vi "energy_optimization_15.vi"() -> ()   [LabVIEW 2016]
uses:
  <vilib>/httpClient/LabVIEWHTTPClient.lvlib
panel:
  out "Battery Output":dbl
  in  "stop":bool
  out "Credits":dbl
  out "Solar+AC+Battery":dbl
  out "Battery":dbl
  in  "Illuminance":dbl
  out "ShutDown":bool
  out "Battery LED":bool
  out "AC LED":bool
  out "Solar LED":bool
  out "AC Output":dbl
  out "Solar Output":dbl
  out "Solar+AC":dbl
  out "Solar Voltage":dbl
  in  "Required":dbl
  out "DC Voltage":dbl
  out "Three Phase Signal":dynamicdata(graph)
  # "OUTPUTS"
  # "INPUTS"
  # "INTERMEDIATE STORAGE"
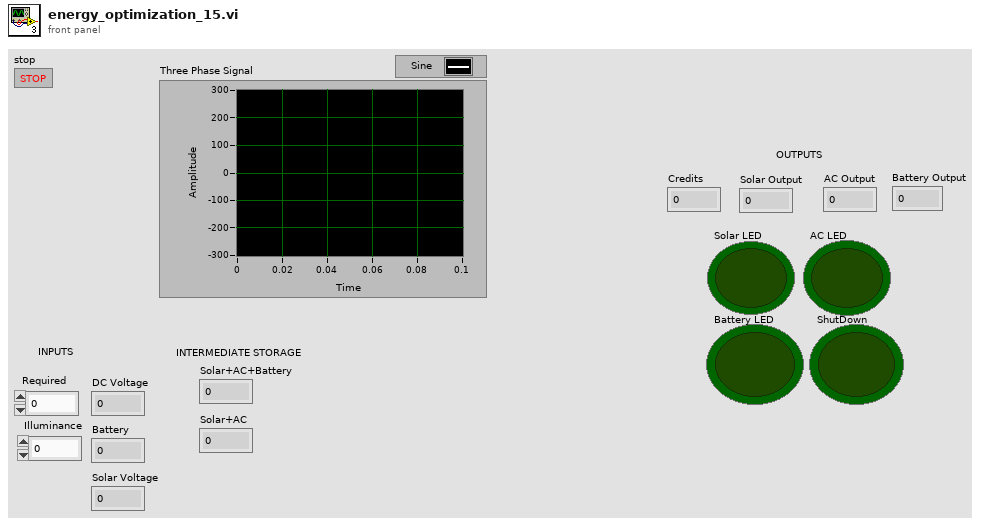
[diagram p1: front panel]
types:
  T1 = typedef "LabVIEWHTTPClient.lvlib/ClientHandle.ctl" = refnum<k1>
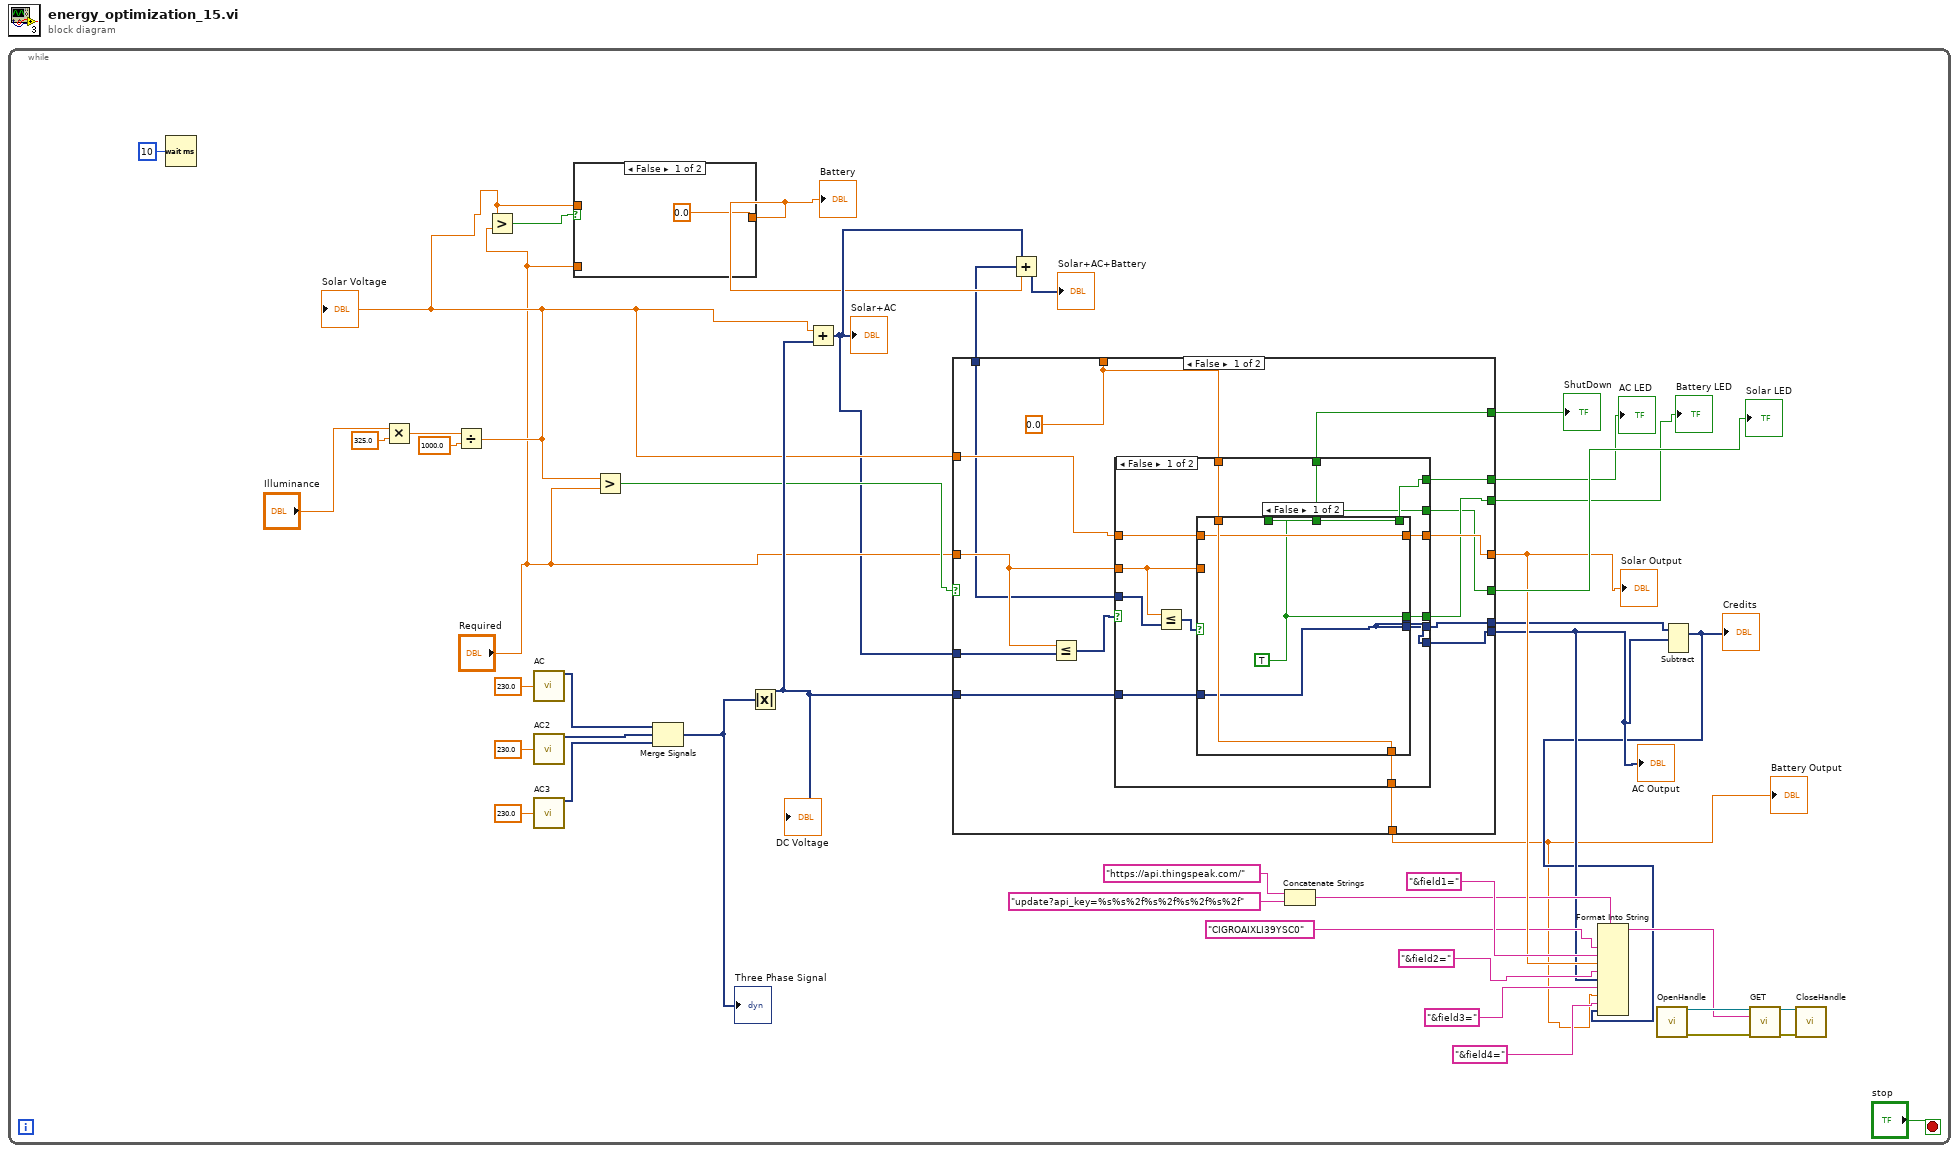
[diagram p0: block diagram]
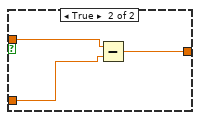
[diagram p2: hidden frame]
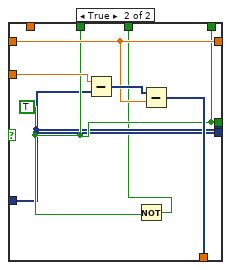
[diagram p3: hidden frame]
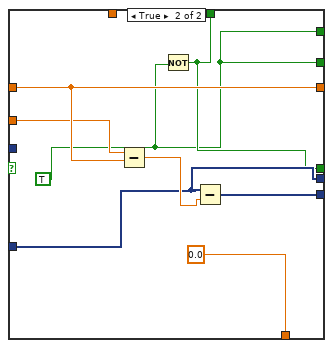
[diagram p4: hidden frame]
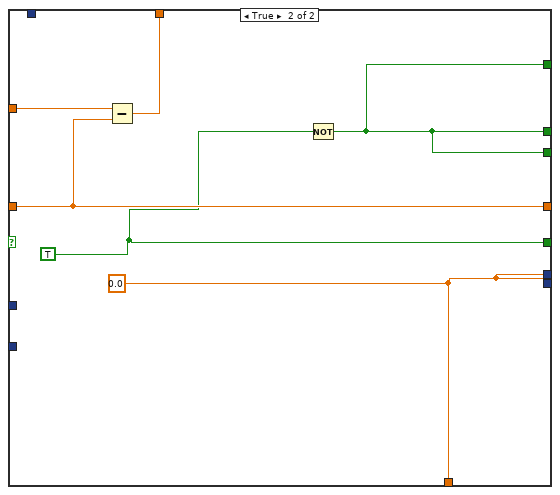
[diagram p5: hidden frame]
diagram:
  n1 = while {
    stop <- "stop" stop-if-true
    n2 = Wait (ms)(milliseconds to wait=u32 10) -> ()  [unwired: 1 out]
    n3 = Multiply(x="Illuminance", y=325.0) -> (x*y=w35:dbl)
    n4 = Divide(x=w35, y=1000.0) -> (x/y=w25:dbl)
    "Solar Voltage" <- w25
    n5 = Greater?(x=w25, y="Required") -> (0:w26:bool)
    n6 = call "AC"("Amplitude"=230.0) -> ("Sine"=w43:dynamicdata)  [unwired: 13 in, 1 out]
    n7 = call "AC2"("Amplitude"=230.0) -> ("Sine"=w42:dynamicdata)  [unwired: 13 in, 1 out]
    n8 = call "AC3"("Amplitude"=230.0) -> ("Sine"=w41:dynamicdata)  [unwired: 13 in, 1 out]
    n9 = case shown="False" w26 {
      tunnel: w25 -> [_ w47]
      tunnel: "Required" -> [_ w46]
      tunnel: [0.0 ("Amplitude") w45] -> w22
      frame False {
      }
      frame True {
        n10 = Subtract(x=w47, y=w46) -> (x-y=w45:dbl)
      }
    }
    "Battery" <- w22
    n11 = Greater?(x=w25, y="Required") -> (0:w28:bool)
    n12 = Merge Signals(w43, w42, w41) -> (w40:dynamicdata)
    "Three Phase Signal" <- w40
    n13 = Absolute Value(x=w40) -> (abs(x)=w29:dynamicdata)
    "DC Voltage" <- w29
    n14 = Add(x=w25, y=w29) -> (x+y=w23:dynamicdata)
    "Solar+AC" <- w23
    n15 = Add(x=w23, y=w22) -> (x+y=w21:dynamicdata)
    "Solar+AC+Battery" <- w21
    n16 = case shown="False" w28 {
      tunnel: [w56 w97] -> w7
      tunnel: [w55 w97] -> w1
      tunnel: [w51 w96] -> w33
      tunnel: [w52 w101] -> w32
      tunnel: [w50 w101] -> w31
      tunnel: [w53 w101] -> w30
      tunnel: w23 -> [w62 _]
      tunnel: "Required" -> [w58 w99]
      tunnel: [w59 w99] -> w12
      tunnel: w25 -> [w60 w100]
      tunnel: [w54 w98] -> _
      tunnel: w29 -> [w57 _]
      tunnel: w21 -> [w49 _]
      tunnel: [w48 w97] -> w6
      frame False {
        w54 = 0.0 ("Amplitude")
        n17 = Less Or Equal?(x=w58, y=w62) -> (x <= y?=w61:dynamicdata)
        n18 = case shown="False" w61 {
          tunnel: w60 -> [w74 w95]
          tunnel: [w73 w95] -> w59
          tunnel: w58 -> [w64 w94]
          tunnel: w57 -> [w75 w90]
          tunnel: [w76 w92] -> w56
          tunnel: [w71 0.0 ("Amplitude")] -> w55
          tunnel: w54 -> [w70 _]
          tunnel: [w67 w89] -> w53
          tunnel: [w69 w88] -> w52
          tunnel: [w68 w88] -> w51
          tunnel: [w66 w89] -> w50
          tunnel: w49 -> [w65 _]
          tunnel: [w63 w90] -> w48
          frame False {
            n19 = Less Or Equal?(x=w64, y=w65) -> (x <= y?=w72:dynamicdata)
            n20 = case shown="False" w72 {
              tunnel: [w77 w82] -> w76
              tunnel: w75 -> [w77 w82]
              tunnel: w74 -> [w79 w85]
              tunnel: [w79 w85] -> w73
              tunnel: w64 -> [_ w87]
              tunnel: [w80 w84] -> w71
              tunnel: w70 -> [w80 _]
              tunnel: [w78 w83] -> w69
              tunnel: [w78 w83] -> w68
              tunnel: [w78 w83] -> w67
              tunnel: [w78 w81] -> w66
              tunnel: [w77 w82] -> w63
              frame False {
                w78 = TRUE
              }
              frame True {
                w83 = TRUE
                n21 = Subtract(x=w87, y=w82) -> (x-y=w86:dynamicdata)
                n22 = Not(x=w83) -> (.not. x?=w81:bool)
                n23 = Subtract(x=w86, y=w85) -> (x-y=w84:dynamicdata)
              }
            }
          }
          frame True {
            w88 = TRUE
            n24 = Subtract(x=w94, y=w95) -> (x-y=w93:dbl)
            n25 = Not(x=w88) -> (.not. x?=w89:bool)
            n26 = Subtract(x=w90, y=w93) -> (x-y=w92:dynamicdata)
          }
        }
      }
      frame True {
        w96 = TRUE
        w97 = 0.0 ("Amplitude")
        n27 = Subtract(x=w100, y=w99) -> (x-y=w98:dbl)
        n28 = Not(x=w96) -> (.not. x?=w101:bool)
      }
    }
    "Solar Output" <- w12
    "AC Output" <- w7
    "Solar LED" <- w33
    "AC LED" <- w32
    "Battery LED" <- w30
    "ShutDown" <- w31
    "Battery Output" <- w1
    n29 = Concatenate Strings("https://api.thingspeak.com/" ("string"), "update?api_key=%s%s%2f%s%2f%s%2f%s%2f" ("string")) -> (w9:string)
    n30 = call <vilib>:"OpenHandle.vi"() -> ("client handle out"=w19:T1, "error out"=w18:errorcluster)  [unwired: 14 in]
    n31 = Subtract(1:w7, 2:w6) -> (0:w3:dynamicdata)  [unwired: 1 in, 1 out]
    "Credits" <- w3
    n32 = Format Into String(format string=w9, "CIGROAIXLI39YSC0" ("string"), "&field1=" ("string"), w12, "&field2=" ("string"), w7, "&field3=" ("string"), w1, "&field4=" ("string"), w3) -> (resulting string=w16:string)  [unwired: 2 in, 1 out]
    n33 = call <vilib>:"GET.vi"("client handle"=w19, "url"=w16, "error in (no error)"=w18) -> ("client handle out"=w20:T1, "error out"=w17:errorcluster)  [unwired: 9 in, 2 out]
    n34 = call <vilib>:"CloseHandle.vi"("client handle"=w20, "error in (no error)"=w17) -> ()  [unwired: 13 in, 1 out]
  }
